vi "niFPGA SGL To U32 Cast.vi"(4 "x":sgl) -> (1 "y":u32)   [LabVIEW 2017]
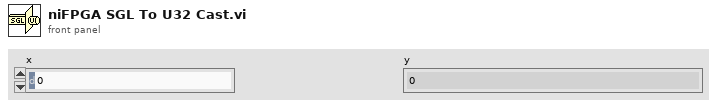
[diagram p1: front panel]
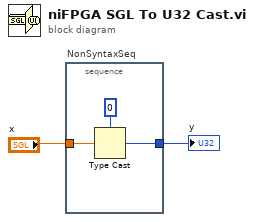
[diagram p0: block diagram]
diagram:
  n1 = stacked-sequence "NonSyntaxSeq" {
    tunnel: "x" -> [w4]
    tunnel: [w3] -> w1
    frame #0 {
      n2 = Type Cast(type=u32 0, x=w4) -> (*(type *) &x=w3:u32)
    }
  }
  "y" <- w1
